vi "List Active Measurements.vi"(8 "error in (no error)":errorcluster, 11 "multicolumnListbox ref in":refnum<vi>) -> (0 "error out":errorcluster, 1 "active measurements list":string[][](array[string]), 2 "active measurement details":T2, 3 "multicolumnListbox ref":refnum<vi>, 4 "create client disabled?":T1(ring))   [LabVIEW 2021, in "Create Measurement Plug-In Client.lvlib"]
uses:
  Create Measurement Plug-In Client.lvlib
  gRPC/Generated APIs/ni/measurementlink/discovery/v1/RPC Messages/ni_measurementlink_discovery_v1_EnumerateServicesResponse.ctl
  gRPC/Generated APIs/ni/measurementlink/discovery/v1/RPC Messages/ni_measurementlink_discovery_v1_ServiceDescriptor.ctl
  gRPC/Generated APIs/ni/measurementlink/discovery/v1/RPC Messages/ni_measurementlink_discovery_v1_ServiceDescriptor_AnnotationsEntry.ctl
  gRPC/Generated APIs/ni/measurementlink/discovery/v1/RPC Messages/ni_measurementlink_discovery_v1_EnumerateServicesRequest.ctl
  Runtime/Clients/Discovery V1/TypeDefs/gRPC Client Cache FGV Action.ctl
  gRPC/Generated APIs/ni/measurementlink/discovery/v1/ni.measurementlink.discovery.v1.api.lvlib
  Runtime/Clients/Discovery V1/NI Discovery V1 Client.lvlib
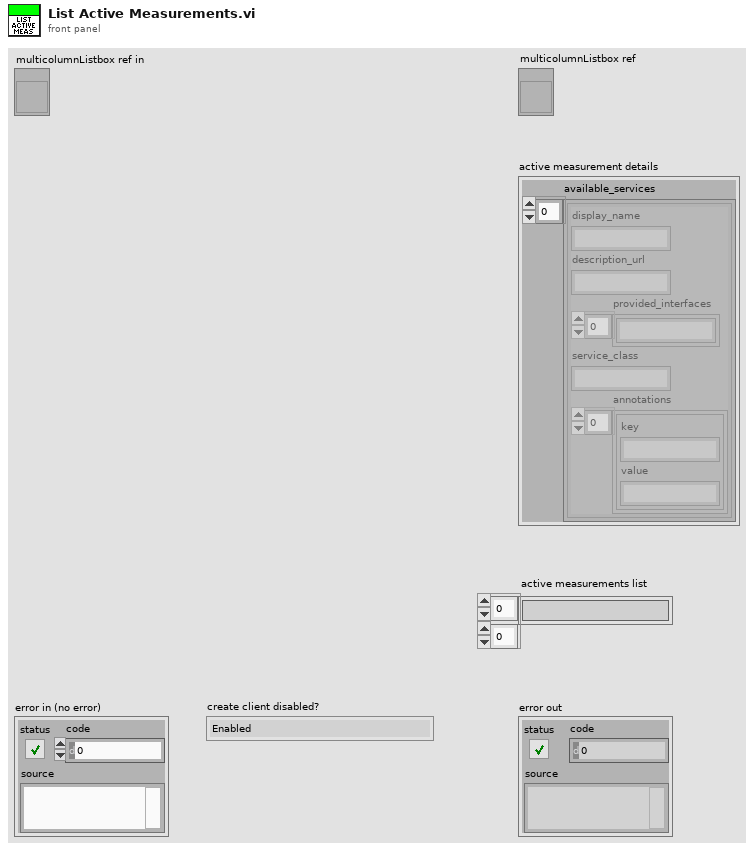
[diagram p1: front panel]
types:
  T1 = enum8{"Enabled", "Disabled", "Disabled and Grayed Out"}
  T2 = typedef "ni.measurementlink.discovery.v1.api.lvlib/ni_measurementlink_discovery_v1_EnumerateServicesResponse.ctl" = cluster{"available_services":T3[]}
  T3 = typedef "ni.measurementlink.discovery.v1.api.lvlib/ni_measurementlink_discovery_v1_ServiceDescriptor.ctl" = cluster{"display_name":string, "description_url":string, "provided_interfaces":string[], "service_class":string, "annotations":T4[]}
  T4 = typedef "ni.measurementlink.discovery.v1.api.lvlib/ni_measurementlink_discovery_v1_ServiceDescriptor_AnnotationsEntry.ctl" = cluster{"key":string, "value":string}
  T5 = typedef "NI Discovery V1 Client.lvlib/gRPC Client Cache FGV Action.ctl" = enum16{"Get Client", "Recreate Client", "Destroy Client", "Update ClusterId"}
  T6 = typedef "ni.measurementlink.discovery.v1.api.lvlib/ni_measurementlink_discovery_v1_EnumerateServicesRequest.ctl" = cluster{"provided_interface":string}
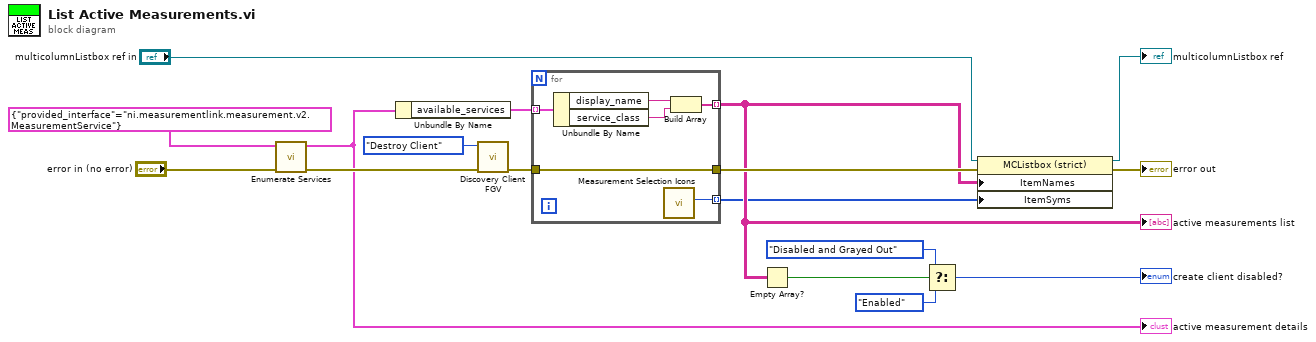
[diagram p0: block diagram]
diagram:
  n1 = call "Enumerate Services.vi"("error in"="error in (no error)", "request data"=T6 {"provided_interface"="ni.measurementlink.measurement.v2.MeasurementService"}) -> ("error out"=w12:errorcluster, "response data"=w2:T2)  [unwired: 7 in]
  "active measurement details" <- w2
  n2 = Unbundle By Name(w2) -> ("available_services"=w10:T3[])
  n3 = call "Discovery Client FGV.vi"("error in"=w12, "action"=gRPC_Client_Cache_FGV_Action."Destroy Client") -> ("error out"=w13:errorcluster)  [unwired: 6 in, 3 out]
  n4 = for {
    tunnel: w10 -> [w20] mode=indexing
    tunnel: [w21] -> w4 mode=indexing
    tunnel: [w18] -> w1 mode=indexing
    tunnel: [w19] -> w14
    tunnel: w13 -> [w19]
    n5 = Unbundle By Name(w20) -> ("display_name"=w23:string, "service_class"=w22:string)
    n6 = call "Measurement Selection Icons.vi"() -> ("Checked"=w18:i32)  [unwired: 10 in, 1 out]
    n7 = Build Array(w23, w22) -> (w21:string[])
  }
  "active measurements list" <- w4
  n8 = Empty Array?(array=w4) -> (empty?=w7:bool)
  n9 = Select(t=T1."Disabled and Grayed Out", s=w7, f=T1."Enabled" ("Disabled")) -> (s? t:f=→"create client disabled?":T1)
  n10 = property class="MCListbox (strict)"(reference="multicolumnListbox ref in", error in=w14, "ItemNames"=w4, "ItemSyms"=w1) -> (reference out=→"multicolumnListbox ref":refnum<vi>, error out=→"error out":errorcluster)
